vi "RSZVB Set Calibration Kit User Connector Type With Label.vi"(7 "Calibration Kit Label (\"\")":string, 8 "error in (no error)":errorcluster {"code" format="%.0x"}, 9 "Calibration Kit Name (\"\")":string, 10 "Connection Type (\"\")":string, 11 "VISA session":refnum<visa-resource-name>) -> (0 "error out":errorcluster {"code" format="%.0x"}, 3 "dup VISA session":refnum<visa-resource-name>)   [LabVIEW 2011]
doc: "Selects the calibration kit to be used, specifying its connector type, name, and label.\n\nRemote-control command(s):\n[SENSe<Ch>:]CORRection:CKIT:LSELect '<conn_type>', '<ckit_name>', '<ckit_label>'"
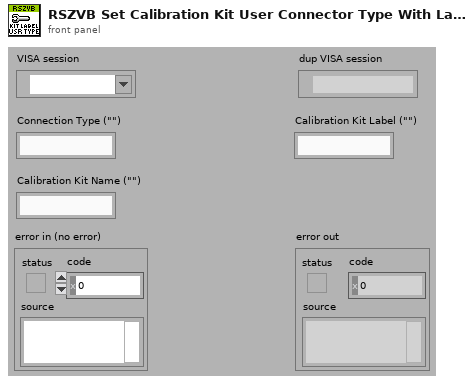
[diagram p1: front panel]
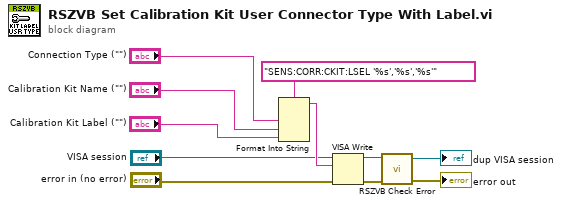
[diagram p0: block diagram]
diagram:
  n1 = Format Into String(format string="SENS:CORR:CKIT:LSEL '%s','%s','%s'", "Connection Type (\"\")", "Calibration Kit Name (\"\")", "Calibration Kit Label (\"\")") -> (resulting string=w8:string)  [unwired: 2 in, 1 out]
  n2 = VISA Write(VISA resource name="VISA session", write buffer=w8, error in (no error)="error in (no error)") -> (VISA resource name out=w10:refnum<visa-resource-name>, error out=w11:errorcluster)  [unwired: 1 out]
  n3 = call "RSZVB Check Error.vi"("error in (no error)"=w11, "VISA session"=w10) -> ("error out"=→"error out":errorcluster, "dup VISA session"=→"dup VISA session":refnum<visa-resource-name>)  [unwired: 8 in]
